vi "Lift Fill Select.vi"(8 "Trigger Buffer":dbl, 10 "Lift Position":dbl, 11 "Config Cluster":T1) -> (3 "Fill Color":dbl)   [LabVIEW 2017]
uses:
  Config Cluster.ctl
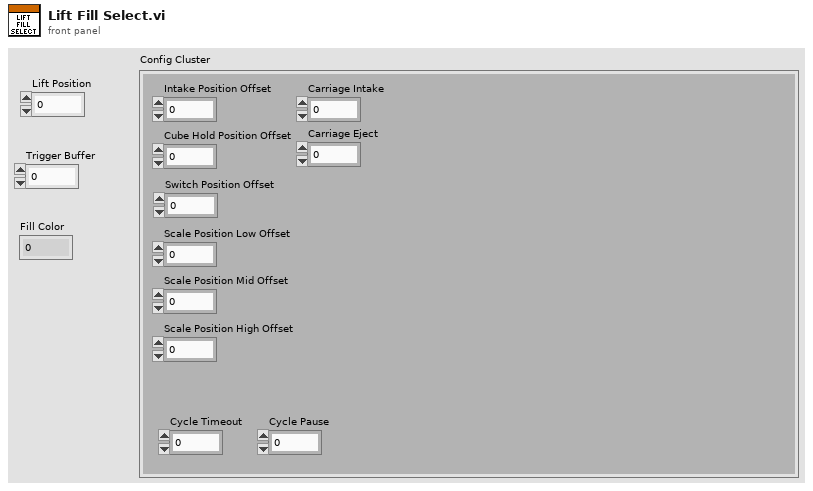
[diagram p1: front panel]
types:
  T1 = typedef "Config Cluster.ctl" = cluster{"Intake Position Offset":dbl, "Cube Hold Position Offset":dbl, "Switch Position Offset":dbl, "Scale Position Low Offset":dbl, "Scale Position Mid Offset":dbl, "Scale Position High Offset":dbl, "Cycle Timeout":dbl, "Cycle Pause":dbl, "Carriage Intake":dbl, "Carriage Eject":dbl}
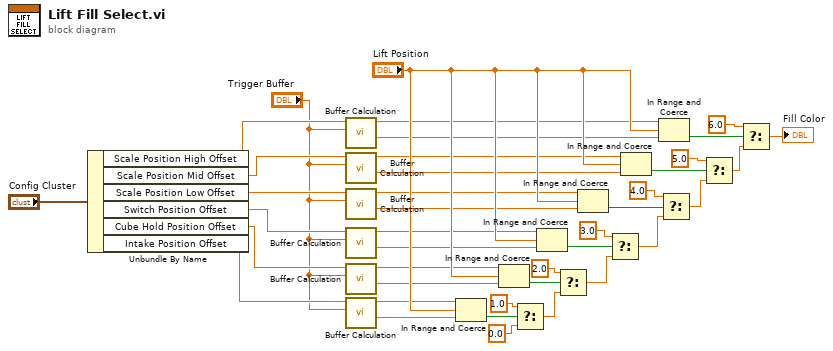
[diagram p0: block diagram]
diagram:
  n1 = Unbundle By Name("Config Cluster") -> ("Scale Position High Offset"=w27:dbl, "Scale Position Mid Offset"=w26:dbl, "Scale Position Low Offset"=w25:dbl, "Switch Position Offset"=w24:dbl, "Cube Hold Position Offset"=w23:dbl, "Intake Position Offset"=w22:dbl)
  n2 = call "Buffer Calculation.vi"("Buffer"="Trigger Buffer", "Input"=w27) -> ("-Buffer"=w37:dbl, "+Buffer"=w38:dbl)  [unwired: 8 in]
  n3 = call "Buffer Calculation.vi"("Buffer"="Trigger Buffer", "Input"=w26) -> ("-Buffer"=w35:dbl, "+Buffer"=w36:dbl)  [unwired: 8 in]
  n4 = call "Buffer Calculation.vi"("Buffer"="Trigger Buffer", "Input"=w25) -> ("-Buffer"=w33:dbl, "+Buffer"=w34:dbl)  [unwired: 8 in]
  n5 = call "Buffer Calculation.vi"("Buffer"="Trigger Buffer", "Input"=w24) -> ("-Buffer"=w31:dbl, "+Buffer"=w32:dbl)  [unwired: 8 in]
  n6 = call "Buffer Calculation.vi"("Buffer"="Trigger Buffer", "Input"=w23) -> ("-Buffer"=w20:dbl, "+Buffer"=w30:dbl)  [unwired: 8 in]
  n7 = call "Buffer Calculation.vi"("Buffer"="Trigger Buffer", "Input"=w22) -> ("-Buffer"=w28:dbl, "+Buffer"=w29:dbl)  [unwired: 8 in]
  n8 = In Range and Coerce(upper limit=w29, x="Lift Position", lower limit=w28) -> (In Range?=w10:bool)  [unwired: 1 out]
  n9 = In Range and Coerce(upper limit=w30, x="Lift Position", lower limit=w20) -> (In Range?=w12:bool)  [unwired: 1 out]
  n10 = Select(t=1.0, s=w10, f=0.0) -> (s? t:f=w9:dbl)
  n11 = In Range and Coerce(upper limit=w32, x="Lift Position", lower limit=w31) -> (In Range?=w13:bool)  [unwired: 1 out]
  n12 = Select(t=2.0, s=w12, f=w9) -> (s? t:f=w11:dbl)
  n13 = In Range and Coerce(upper limit=w34, x="Lift Position", lower limit=w33) -> (In Range?=w15:bool)  [unwired: 1 out]
  n14 = Select(t=3.0, s=w13, f=w11) -> (s? t:f=w14:dbl)
  n15 = In Range and Coerce(upper limit=w36, x="Lift Position", lower limit=w35) -> (In Range?=w17:bool)  [unwired: 1 out]
  n16 = In Range and Coerce(upper limit=w38, x="Lift Position", lower limit=w37) -> (In Range?=w19:bool)  [unwired: 1 out]
  n17 = Select(t=4.0, s=w15, f=w14) -> (s? t:f=w16:dbl)
  n18 = Select(t=5.0, s=w17, f=w16) -> (s? t:f=w18:dbl)
  n19 = Select(t=6.0, s=w19, f=w18) -> (s? t:f=→"Fill Color":dbl)
